vi "Untitled 2.vi"() -> ()   [LabVIEW 2020]
panel:
  out "Waveform Chart":i32[](graph)
  out "size(s)":i32
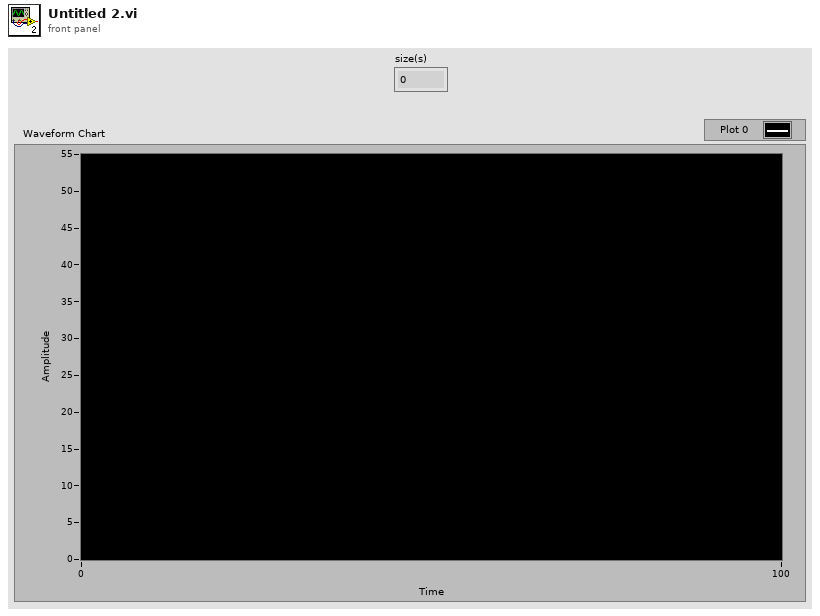
[diagram p1: front panel]
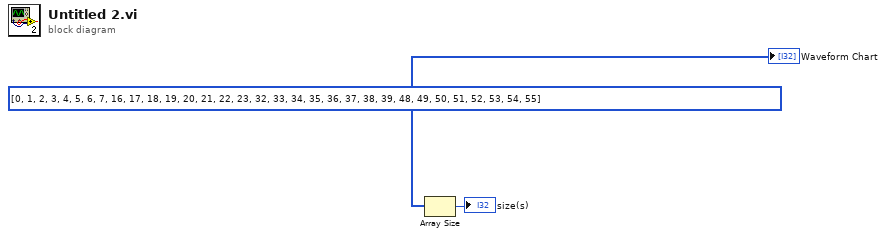
[diagram p0: block diagram]
diagram:
  w1 = i32[] [0, 1, 2, 3, 4, 5, 6, 7, 16, 17, 18, 19, 20, 21, 22, 23, 32, 33, 34, 35, 36, 37, 38, 39, 48, 49, 50, 51, 52, 53, 54, 55]
  n1 = Array Size(array=w1) -> (size(s)=→"size(s)":i32)
  "Waveform Chart" <- w1
